vi "Visualize Found Peak.vi"(8 "error in (no error)":errorcluster, 10 "Found Peak":refnum<data-value>, 11 "Application Manager in":refnum<class "Application Manager.lvclass">) -> (0 "error out":errorcluster, 3 "Application Manager out":refnum<class "Application Manager.lvclass">)   [LabVIEW 2025, in "Application Manager.lvlib" / "Application Manager.lvclass"]
uses:
  Application Manager.lvclass
  Application Manager.lvclass/Application Manager.ctl
  UI/UI Root/UI Root Messages/Visualise found peak Msg/Visualise found peak Msg.lvclass/Visualise found peak Msg.ctl
  <vilib>/ActorFramework/Message Enqueuer/Message Enqueuer.lvclass/Message Enqueuer.ctl
  <vilib>/ActorFramework/Message Enqueuer/Enqueue.vi
  UI/UI Root/UI Root Messages/Visualise found peak Msg/Visualise found peak Msg.lvclass
  <vilib>/ActorFramework/Message Priority Queue/Priority Enqueue.vi
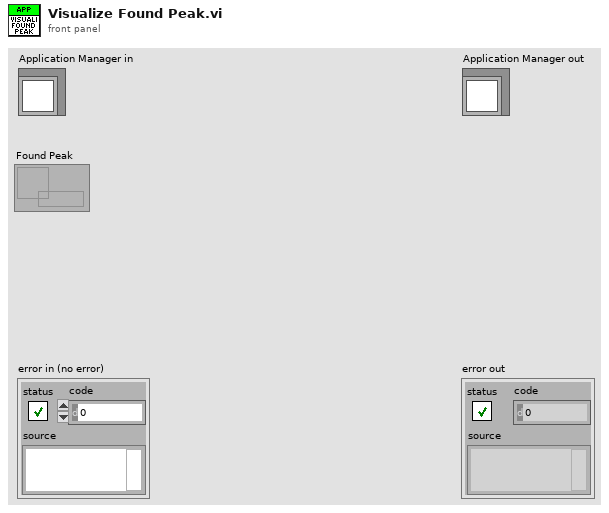
[diagram p1: front panel]
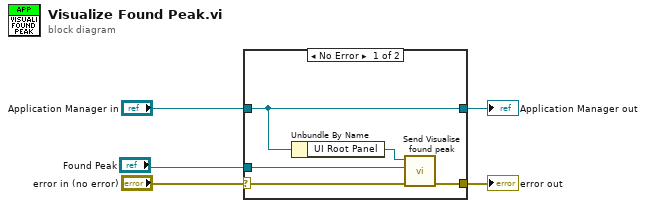
[diagram p0: block diagram]
diagram:
  n1 = case shown="No Error" "error in (no error)" {
    selector: "error in (no error)" -> [w7 w12]
    tunnel: [w6 w12] -> w4
    tunnel: [w10 w11] -> w2
    tunnel: "Application Manager in" -> [w10 w11]
    tunnel: "Found Peak" -> [w8 _]
    frame No Error {
      n2 = Unbundle By Name(w10) -> ("UI Root Panel"=w9:refnum<class "Message Enqueuer.lvclass">)
      n3 = call "Send Visualise found peak.vi"("error in (no error)"=w7, "Found Peak"=w8, "Message Enqueuer"=w9) -> ("error out"=w6:errorcluster)  [unwired: 7 in, 1 out]
    }
    frame Error {
    }
  }
  "error out" <- w4
  "Application Manager out" <- w2
